vi "Clockwiselogic.vi"(8 "error in (no error)":errorcluster, 11 "Programming Logic in":refnum<class "Programming Logic.lvclass">) -> (0 "error out":errorcluster, 3 "Programming Logic out":refnum<class "Programming Logic.lvclass">)   [LabVIEW 2014, in "Files Library.lvlib" / "Programming Logic.lvclass"]
uses:
  Programming Logic.lvclass
  Programming Logic.lvclass/Programming Logic.ctl
  Files Library.lvlib
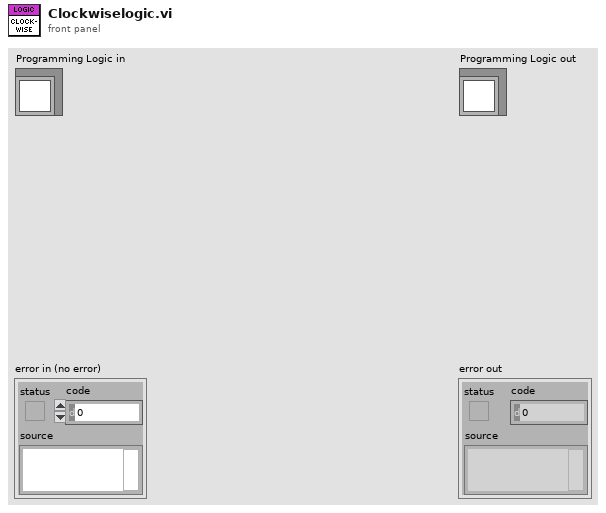
[diagram p1: front panel]
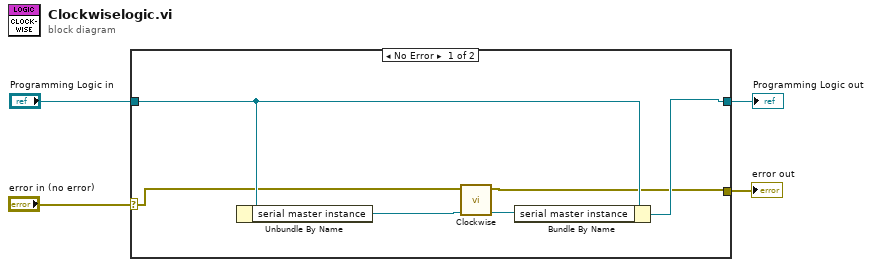
[diagram p0: block diagram]
diagram:
  n1 = case shown="No Error" "error in (no error)" {
    selector: "error in (no error)" -> [w6 w12]
    tunnel: [w5 w12] -> w3
    tunnel: [w7 w11] -> w1
    tunnel: "Programming Logic in" -> [w9 w11]
    frame No Error {
      n2 = Unbundle By Name(w9) -> ("serial master instance"=w10:refnum<class "Modbus Master.lvclass">)
      n3 = call "Clockwise.vi"("Modbus instance in"=w10, "error in"=w6) -> ("Modbus instance out"=w8:refnum<class "Modbus Master.lvclass">, "error out"=w5:errorcluster)  [unwired: 8 in]
      n4 = Bundle By Name(cluster=w9, "serial master instance"=w8) -> (w7:refnum<class "Programming Logic.lvclass">)
    }
    frame Error {
    }
  }
  "error out" <- w3
  "Programming Logic out" <- w1
